vi "Tabla de multiplicar.vi"() -> ()   [LabVIEW 2016]
panel:
  out "resultado":dbl
  out "tablas de multiplicar":dbl[][](array[numeric])
  in  "num 2":dbl
  in  "num 1":dbl
  in  "renglones":dbl
  in  "columnas":dbl
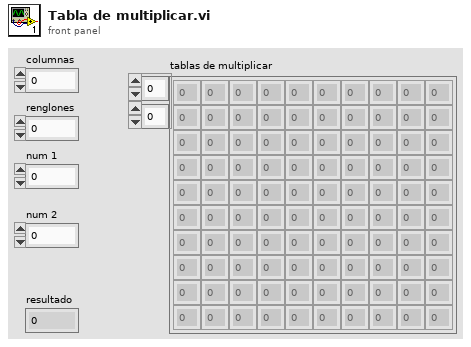
[diagram p1: front panel]
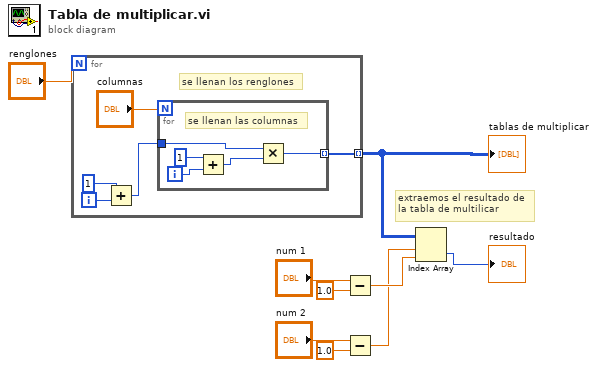
[diagram p0: block diagram]
diagram:
  # "extraemos el resultado de\nla tabla de multilicar"
  n1 = for {
    N: "renglones" -> [_]
    tunnel: [w11] -> w8 mode=indexing
    i -> [w14]
    # "se llenan los renglones"
    n2 = Add(x=1, y=w14) -> (x+y=w12:i32)
    n3 = for {
      N: "columnas" -> [_]
      tunnel: w12 -> [w16]
      tunnel: [w15] -> w11 mode=indexing
      i -> [w19]
      # "se llenan las columnas"
      n4 = Add(x=1, y=w19) -> (x+y=w17:i32)
      n5 = Multiply(x=w16, y=w17) -> (x*y=w15:i32)
    }
  }
  "tablas de multiplicar" <- w8
  n6 = Subtract(x="num 1", y=1.0) -> (x-y=w3:dbl)
  n7 = Subtract(x="num 2", y=1.0) -> (x-y=w2:dbl)
  n8 = Index Array(array=w8, index (row)=w2, index (col)=w3) -> (element=→"resultado":i32)
